vi "CRYPEAQ exIndex.vi"(11 "f":dbl[](array[numeric])) -> (3 "s(Excitation index)":dbl[](array[numeric]))   [LabVIEW 2013]
panel:
  out "XY Graph 2":cluster{"Center Frequency":dbl[], dbl[]}(graph)
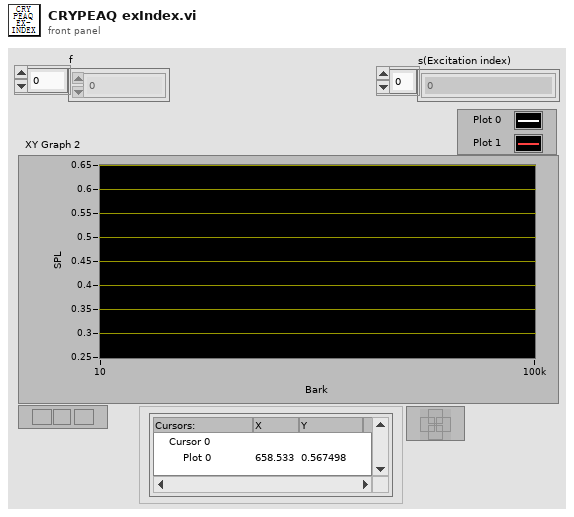
[diagram p1: front panel]
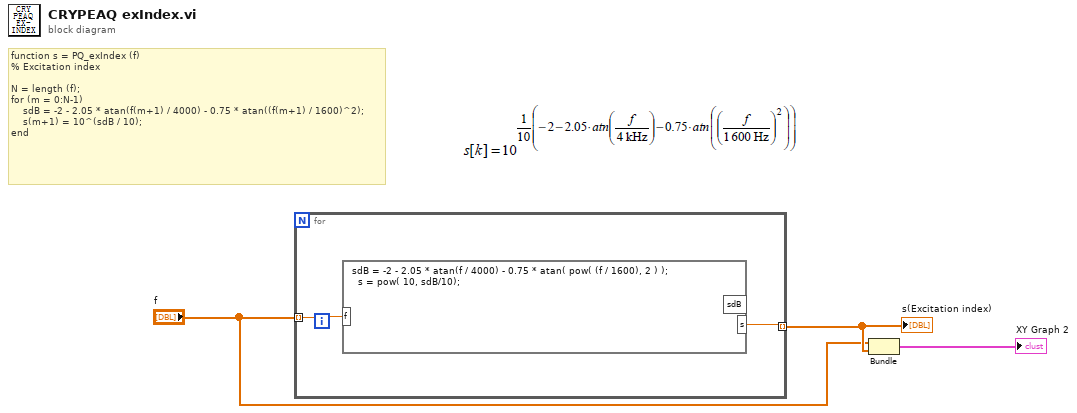
[diagram p0: block diagram]
diagram:
  # "function s = PQ_exIndex (f)\n% Excitation index\n\nN = length (f);\nfor (m = 0:N-1)\n    sdB = -2 - 2.05 * atan(f(m+1) / 4000) - 0.75 * atan((f(m+1) / 1600)^2);\n    s(m+1) = 10^(sdB / 10);\nend"
  n1 = for {
    tunnel: "f" -> [w5] mode=indexing
    tunnel: [w4] -> w3 mode=indexing
    n2 = formula code="sdB = -2 - 2.05 * atan(f / 4000) - 0.75 * atan( pow( (f / 1600), 2 ) );\n  s = pow( 10, sdB/10);"("f"=w5) -> ("s"=w4:dbl)  [unwired: 1 out]
  }
  "s(Excitation index)" <- w3
  n3 = Bundle("f"="f", w3) -> (→"XY Graph 2":cluster{"f":dbl[], dbl[]})  [unwired: 1 in]
